vi "readDefaultValuesFromDisk.vi"(1 "appFolder":path, 5 "error in (no error)":errorcluster, 7 "Control Label":string, 9 "Caption":string) -> (13 "Value (XML String)":string, 15 "appFolder DUMP":path, 19 "error out":errorcluster)   [LabVIEW 2022 SP3, in "stillnessHelper.lvclass"]
uses:
  stillnessHelper.lvclass
  <userlib>/_OpenG.lib/file/file.llb/File Exists - Scalar__ogtk.vi
  <vilib>/Utility/xml.llb/Read From XML File(string).vi
  <userlib>/_OpenG.lib/file/file.llb/openg_file.lvlib
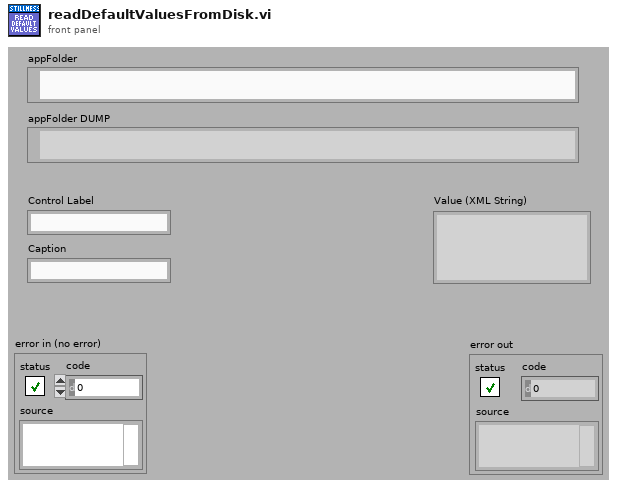
[diagram p1: front panel]
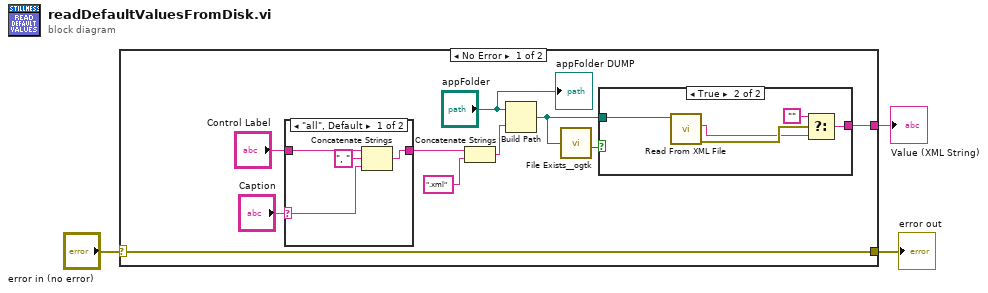
[diagram p0: block diagram]
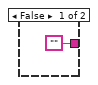
[diagram p3: hidden frame]
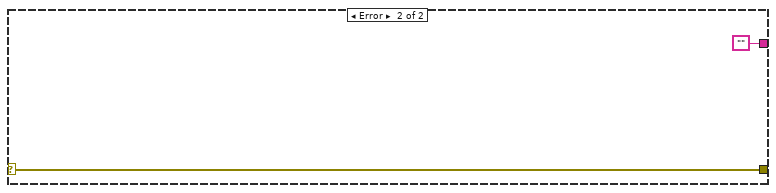
[diagram p4: hidden frame]
diagram:
  n1 = case shown="No Error" "error in (no error)" {
    selector: "error in (no error)" -> [w6 w26]
    tunnel: [w6 w26] -> w2
    tunnel: [w7 ""] -> w1
    frame No Error {
      n2 = case shown="\"all\", Default" "Caption" {
        selector: "Caption" -> [w14 _]
        tunnel: [w17 w18] -> w10
        tunnel: "Control Label" -> [w16 w18]
        frame "all", Default {
          n3 = Concatenate Strings(w16, ", " ("string"), w14) -> (w17:string)
        }
        frame "" {
        }
      }
      n4 = Concatenate Strings(w10, ".xml" ("string")) -> (w12:string)
      n5 = Build Path(base path="appFolder", name or relative path=w12) -> (appended path=w4:path)
      n6 = call-poly <userlib>:"File Exists__ogtk.vi"("file path"=w4) -> ("exists"=w8:bool)  [unwired: 6 in, 1 out]
      n7 = case shown="True" w8 {
        tunnel: w4 -> [_ w24]
        tunnel: ["" w21] -> w7
        frame False {
        }
        frame True {
          n8 = call-poly <vilib>:"Read From XML File.vi"("XML File Path"=w24) -> ("error out"=w23:errorcluster, "XML Elements"=w22:string)  [unwired: 8 in, 1 out]
          n9 = Select(t="", s=w23, f=w22) -> (s? t:f=w21:string)
        }
      }
      "appFolder DUMP" <- "appFolder"
    }
    frame Error {
    }
  }
  "error out" <- w2
  "Value (XML String)" <- w1
